vi "Parse Adaptor Info.vi"(8 "error in (no error)":errorcluster, 11 "Adaptor Info XML":string="<?xml version=\"1.0\" encoding=\"UTF-8\"?><ns2:tooladapter xmlns:ns2=\"http://jazz.net/xmlns/alm/qm/v0.1/\" xmlns:ns1=\"http://schema.ibm.com/vega/2008/\" xmlns:ns3=\"http://purl.org/dc/elements/1.1/\" xmlns:ns4=\"http://jazz.net/xmlns/prod/jazz/process/0.6/\" xmlns:ns5=\"http://jazz.net/xmlns/alm/v0.1/\" xmlns:ns6=\"http://www.w3.org/1999/02/22-rdf-syntax-ns#\" xmlns:ns7=\"http://purl.org/dc/terms/\" xmlns:ns8=\"http://jazz.net/xmlns/alm/qm/v0.1/tsl/v0.1/\" xmlns:ns9=\"http://jazz.net/xmlns/alm/qm/v0.1/testscript/v0.1/\" xmlns:ns10=\"http://jazz.net/xmlns/alm/qm/qmadapter/task/v0.1\" xmlns:ns11=\"http://jazz.net/xmlns/alm/qm/qmadapter/v0.1\" xmlns:ns12=\"http://jazz.net/xmlns/alm/qm/v0.1/executionworkitem/v0.1\" xmlns:ns13=\"http://jazz.net/xmlns/alm/qm/v0.1/executionresult/v0.1\" xmlns:ns14=\"http://jazz.net/xmlns/alm/qm/v0.1/catalog/v0.1\" xmlns:ns16=\"http://jazz.net/xmlns/alm/qm/styleinfo/v0.1/\" xmlns:ns17=\"http://www.w3.org/1999/XSL/Transform\"><ns2:projectArea alias=\"JKE+Banking+%28Quality+Management%29\" href=\"https://10.144.10.217:9443/qm/resource/itemOid/com.ibm.team.process.ProjectArea/_uAKaoJnNEeKUYIkbmzCY0Q\"/><ns3:identifier>https://10.144.10.217:9443/qm/service/com.ibm.rqm.integration.service.IIntegrationService/resources/JKE+Banking+%28Quality+Management%29/adapter/myAdaptorID</ns3:identifier><ns2:webId>3</ns2:webId><ns3:title>myAdaptorName</ns3:title><ns3:description>myDescription</ns3:description><ns3:creator ns6:resource=\"https://10.144.10.217:9443/jts/resource/itemName/com.ibm.team.repository.Contributor/zhonghaijun\">zhonghaijun</ns3:creator><ns11:type>com.ni.rqm.adapter</ns11:type><ns11:pollinginterval>5000</ns11:pollinginterval><ns11:lastheartbeat>1367329580085</ns11:lastheartbeat><ns11:hostname>LVL-Gregm</ns11:hostname><ns11:ipaddress>10.0.43.157</ns11:ipaddress><ns11:macaddress>00-FF-A0-B3-26-06</ns11:macaddress><ns11:fqdn>LVL-Gregm.amer.corp.natinst.com</ns11:fqdn><ns11:capability>EXECUTE</ns11:capability><ns11:capability>IMPORT</ns11:capability><ns11:instructions href=\"https://10.144.10.217:9443/qm/service/com.ibm.rqm.integration.service.IIntegrationService/resources/JKE+Banking+%28Quality+Management%29/instructions/myAdaptorID\"/><ns11:tasks href=\"https://10.144.10.217:9443/qm/service/com.ibm.rqm.integration.service.IIntegrationService/resources/JKE+Banking+%28Quality+Management%29/tasks?adapterId=myAdaptorID\"/></ns2:tooladapter>") -> (0 "error out":errorcluster, 2 "Tasks URL":string, 3 "Instructions URL":string)   [LabVIEW 2012]
uses:
  <vilib>/xml/Load XML String.vi
  <vilib>/xml/Close Reference(Node).vi
  <vilib>/xml/Close Reference(NNMap).vi
  <vilib>/xml/Close Reference(NdList).vi
  <vilib>/xml/NI_XML.lvlib
  <resource>/objmgr/DOMUserDefRef.rc
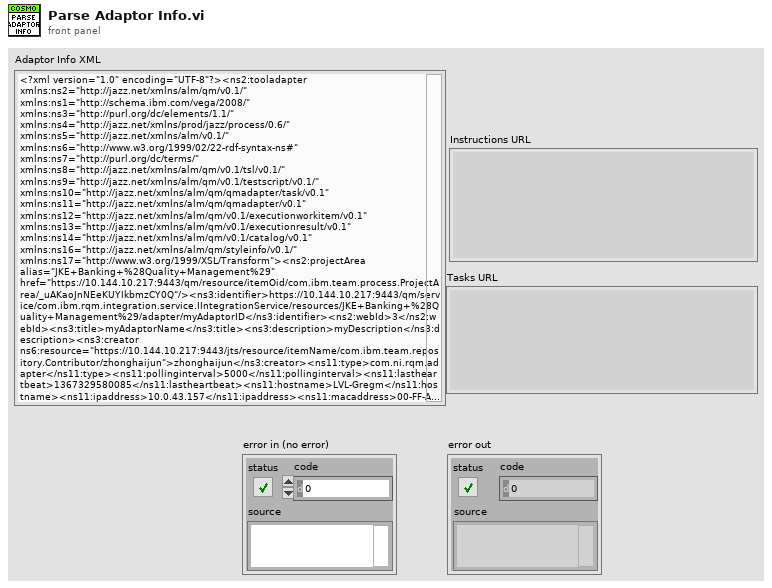
[diagram p1: front panel]
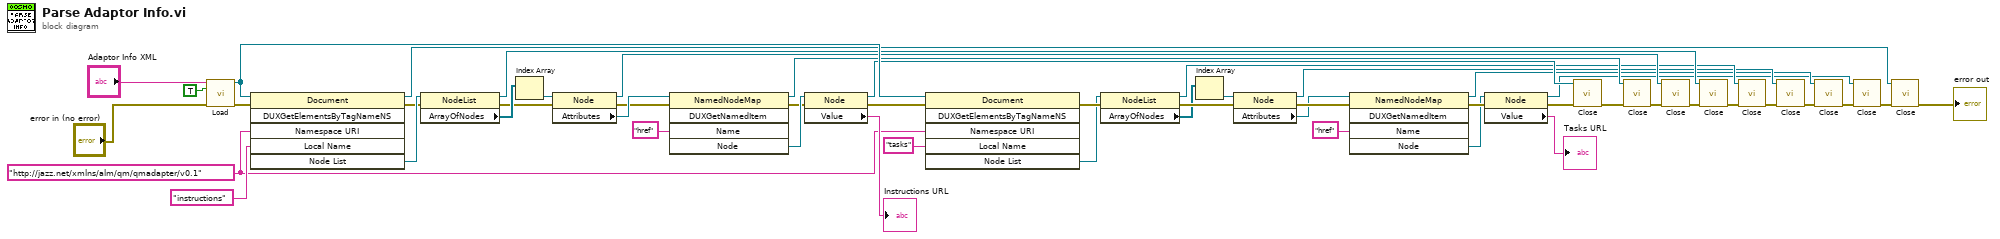
[diagram p0: block diagram]
diagram:
  w23 = "http://jazz.net/xmlns/alm/qm/qmadapter/v0.1" ("Namespace URI")
  n1 = call-poly <vilib>:"Load.vi"("XML string"="Adaptor Info XML", "process namespaces (False)"=TRUE, "error in (no error)"="error in (no error)") -> ("DOM document out"=w25:refnum<k20>, "error out"=w45:errorcluster)  [unwired: 10 in, 1 out]
  n2 = invoke class="Document" method="DUXGetElementsByTagNameNS"(reference=w25, error in=w45, "Namespace URI"=w23, "Local Name"="instructions") -> (reference out=w12:refnum<k20>, error out=w46:errorcluster, "Node List"=w47:refnum<k20>)  [unwired: 2 in, 3 out]
  n3 = property class="NodeList"(reference=w47, error in=w46) -> (reference out=w14:refnum<k20>, error out=w38:errorcluster, "ArrayOfNodes"=w44:refnum<k20>[])
  n4 = Index Array(array=w44) -> (element=w43:refnum<k20>)  [unwired: 1 in]
  n5 = property class="Node"(reference=w43, error in=w38) -> (reference out=w15:refnum<k20>, error out=w37:errorcluster, "Attributes"=w42:refnum<k20>)
  n6 = invoke class="NamedNodeMap" method="DUXGetNamedItem"(reference=w42, error in=w37, "Name"="href") -> (reference out=w18:refnum<k20>, error out=w36:errorcluster, "Node"=w40:refnum<k20>)  [unwired: 2 in, 2 out]
  n7 = property class="Node"(reference=w40, error in=w36) -> (reference out=w20:refnum<k20>, error out=w24:errorcluster, "Value"=→"Instructions URL":string)
  n8 = invoke class="Document" method="DUXGetElementsByTagNameNS"(reference=w25, error in=w24, "Namespace URI"=w23, "Local Name"="tasks") -> (error out=w27:errorcluster, "Node List"=w26:refnum<k20>)  [unwired: 2 in, 4 out]
  n9 = property class="NodeList"(reference=w26, error in=w27) -> (reference out=w11:refnum<k20>, error out=w33:errorcluster, "ArrayOfNodes"=w28:refnum<k20>[])
  n10 = Index Array(array=w28) -> (element=w29:refnum<k20>)  [unwired: 1 in]
  n11 = property class="Node"(reference=w29, error in=w33) -> (reference out=w10:refnum<k20>, error out=w34:errorcluster, "Attributes"=w30:refnum<k20>)
  n12 = invoke class="NamedNodeMap" method="DUXGetNamedItem"(reference=w30, error in=w34, "Name"="href") -> (reference out=w9:refnum<k20>, error out=w35:errorcluster, "Node"=w32:refnum<k20>)  [unwired: 2 in, 2 out]
  n13 = property class="Node"(reference=w32, error in=w35) -> (reference out=w3:refnum<k20>, error out=w19:errorcluster, "Value"=→"Tasks URL":string)
  n14 = call-poly <vilib>:"Close.vi"("error in (no error)"=w19, "node"=w20) -> ("error out"=w17:errorcluster)  [unwired: 7 in]
  n15 = call-poly <vilib>:"Close.vi"("error in (no error)"=w17, "named node map"=w18) -> ("error out"=w16:errorcluster)  [unwired: 7 in]
  n16 = call-poly <vilib>:"Close.vi"("error in (no error)"=w16, "node"=w15) -> ("error out"=w13:errorcluster)  [unwired: 7 in]
  n17 = call-poly <vilib>:"Close.vi"("error in (no error)"=w13, "node list"=w14) -> ("error out"=w8:errorcluster)  [unwired: 7 in]
  n18 = call-poly <vilib>:"Close.vi"("error in (no error)"=w8, "node list"=w11) -> ("error out"=w7:errorcluster)  [unwired: 7 in]
  n19 = call-poly <vilib>:"Close.vi"("error in (no error)"=w7, "node"=w10) -> ("error out"=w6:errorcluster)  [unwired: 7 in]
  n20 = call-poly <vilib>:"Close.vi"("error in (no error)"=w6, "named node map"=w9) -> ("error out"=w5:errorcluster)  [unwired: 7 in]
  n21 = call-poly <vilib>:"Close.vi"("error in (no error)"=w5, "node"=w3) -> ("error out"=w4:errorcluster)  [unwired: 7 in]
  n22 = call-poly <vilib>:"Close.vi"("error in (no error)"=w4, "node"=w12) -> ("error out"=→"error out":errorcluster)  [unwired: 7 in]
